vi "Write Numeric Control.vi"(8 "error in (no error)":errorcluster, 10 "Numeric Control":dbl, 11 "ParentClass in":refnum<class "ParentClass.lvclass">) -> (0 "error out":errorcluster, 3 "ParentClass out":refnum<class "ParentClass.lvclass">)   [LabVIEW 2012, in "ParentClass.lvclass"]
uses:
  ParentClass.lvclass
  ParentClass.lvclass/ParentClass.ctl
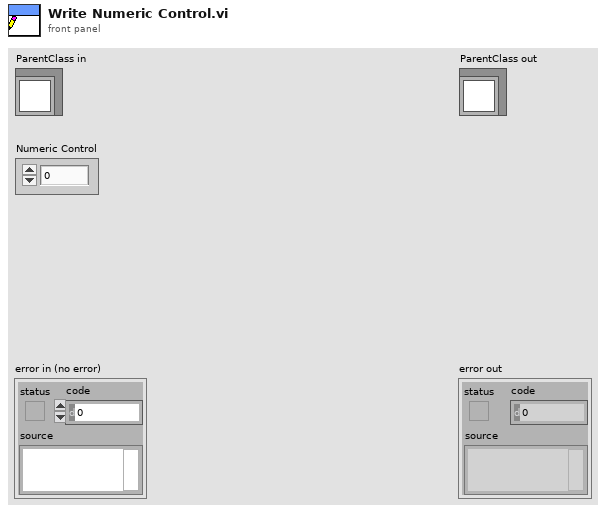
[diagram p1: front panel]
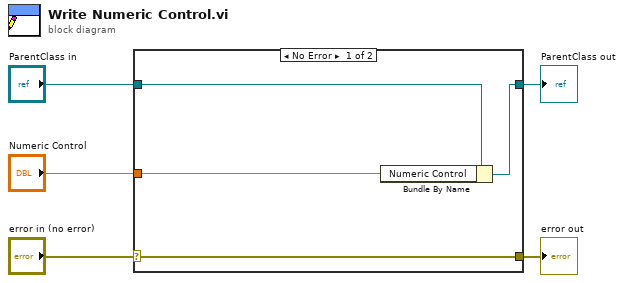
[diagram p0: block diagram]
diagram:
  n1 = case shown="No Error" "error in (no error)" {
    selector: "error in (no error)" -> [w9 w10]
    tunnel: [w9 w10] -> w4
    tunnel: [w7 w11] -> w2
    tunnel: "ParentClass in" -> [w8 w11]
    tunnel: "Numeric Control" -> [w6 _]
    frame No Error {
      n2 = Bundle By Name(cluster=w8, "Numeric Control"=w6) -> (w7:refnum<class "ParentClass.lvclass">)
    }
    frame Error {
    }
  }
  "error out" <- w4
  "ParentClass out" <- w2
